vi "Global CTRL VELOCITA.vi"() -> ()   [LabVIEW 2019]
panel:
  out "CRTL VELOCITA":bool
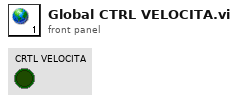
[diagram p1: front panel]
diagram:
